vi "Remove Child.vi"(8 "error in (no error)":errorcluster, 10 "Child":refnum<class "Config Element.lvclass">, 11 "Config Element in":refnum<class "Config Element.lvclass">) -> (0 "error out":errorcluster, 3 "Config Element out":refnum<class "Config Element.lvclass">)   [LabVIEW 2023, in "CDM-Config.lvlib" / "Config Element.lvclass"]
doc: "Removes a child element from this element. If the specified <b>Child</b> is not a direct child of this element, and error is returned."
uses:
  Config Element.lvclass
  Config Element.lvclass/Config Element.ctl
  Config Manager/Config Manager.lvclass
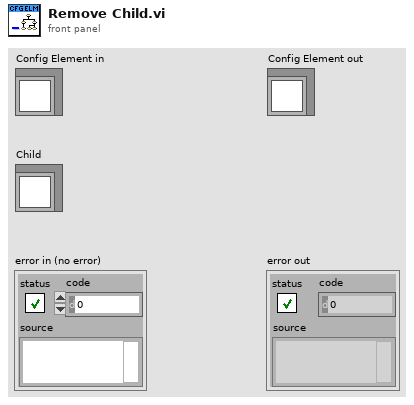
[diagram p1: front panel]
types:
  T1 = typedef "CDM-Config.lvlib/Config Element.lvclass/Element Data.ctl" = cluster{"Node Info":T2, "Owner":refnum<class>, "Changed":bool, "Name":string, "Meta Data":T3[], "Value Type":T4, "Value":variant}
  T2 = typedef "CDM-Config.lvlib/Node Info.ctl" = cluster{"Index":i32, "Parent":i32, "Children":i32[]}
  T3 = typedef "CDM-Config.lvlib/Meta Data.ctl" = cluster{"Name":string, "Value":string}
  T4 = typedef "CDM-Config.lvlib/Value Type.ctl" = enum16{"String", "Number", "Bool", "Object", "Array"}
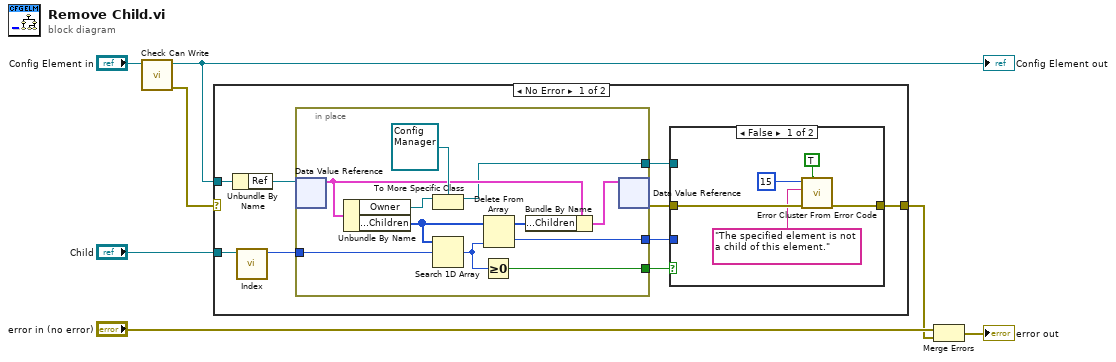
[diagram p0: block diagram]
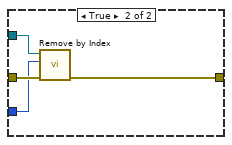
[diagram p2: hidden frame]
diagram:
  n1 = call "Check Can Write.vi"("Config Element in"="Config Element in") -> ("error out"=w1:errorcluster, "Config Element out"=w2:refnum<class "Config Element.lvclass">)  [unwired: 9 in]
  "Config Element out" <- w2
  n2 = case shown="No Error" w1 {
    selector: w1 -> [_ w37]
    tunnel: "Child" -> [w16 _]
    tunnel: w2 -> [w14 _]
    tunnel: [w8 w37] -> w3
    frame No Error {
      n3 = Unbundle By Name(w14) -> ("Ref"=w15:refnum<data-value>)
      n4 = call "Index.vi"("Config Element in"=w16) -> ("Index"=w13:i32)  [unwired: 9 in, 1 out]
      n5 = in-place {
        in-place-border: w13 -> [w36]
        in-place-border: [w31] -> w11
        in-place-border: [w27] -> w10
        in-place-border: [w26] -> w12
        n6 = in-place-dvr #1(w15) -> (w30:T1)  [unwired: 1 out]
        n7 = Unbundle By Name(w30) -> ("Owner"=w33:refnum<class>, "Node Info.Children"=w34:i32[])
        n8 = To More Specific Class(target class=refnum<class "Config Manager.lvclass"> refnum ("CDM-Config.lvlib:Config Manager.lvclass"), reference=w33) -> (specific class reference=w27:refnum<class "Config Manager.lvclass">)  [unwired: 1 in, 1 out]
        n9 = Search 1D Array(1D array=w34, element=w36) -> (index of element=w35:i32)  [unwired: 1 in]
        n10 = Greater Or Equal To 0?(x=w35) -> (x >= 0?=w26:bool)
        n11 = Delete From Array(array=w34, index=w35) -> (deleted portion=w31:i32, array with subset deleted=w29:i32[])  [unwired: 1 in]
        n12 = Bundle By Name(cluster=w30, "Node Info.Children"=w29) -> (w28:T1)
        n13 = in-place-dvr #1(w28) -> (w9:errorcluster)  [unwired: 1 out]
      }
      n14 = case shown="False" w12 {
        tunnel: w11 -> [_ w23]
        tunnel: w10 -> [_ w24]
        tunnel: w9 -> [w21 w25]
        tunnel: [w20 w22] -> w8
        frame False {
          n15 = call <vilib>:"Error Cluster From Error Code.vi"("show call chain? (False)"=TRUE, "error in (no error)"=w21, "error message (\"\")"="The specified element is not a child of this element.", "error code (0)"=15) -> ("error out"=w20:errorcluster)  [unwired: 5 in]
        }
        frame True {
          n16 = call "Remove by Index.vi"("error in (no error)"=w25, "Index"=w23, "Config Manager in"=w24) -> ("error out"=w22:errorcluster)  [unwired: 7 in, 1 out]
        }
      }
    }
    frame Error {
    }
  }
  n17 = Merge Errors("error in (no error)", w3) -> (→"error out":errorcluster)
